vi "TdmsIcons_WriteIcon.vi"(8 "error in (no error)":errorcluster, 9 "Icon":T1, 10 "Function":string="Add", 11 "TdmsIn":refnum<k34>) -> (0 "error out":errorcluster, 3 "TdmsOut":refnum<k34>)   [LabVIEW 2014]
uses:
  <vilib>/picture/picture.llb/imagedata.ctl
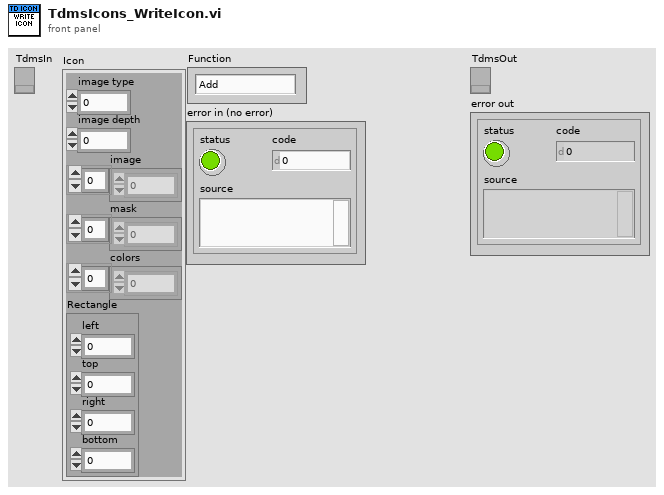
[diagram p1: front panel]
types:
  T1 = typedef "imagedata.ctl" = cluster{"image type":i32, "image depth":i32, "image":u8[], "mask":u8[], "colors":u32[], "Rectangle":cluster{"left":i16, "top":i16, "right":i16, "bottom":i16}}
  T2 = cluster{"left":i16, "top":i16, "right":i16, "bottom":i16}
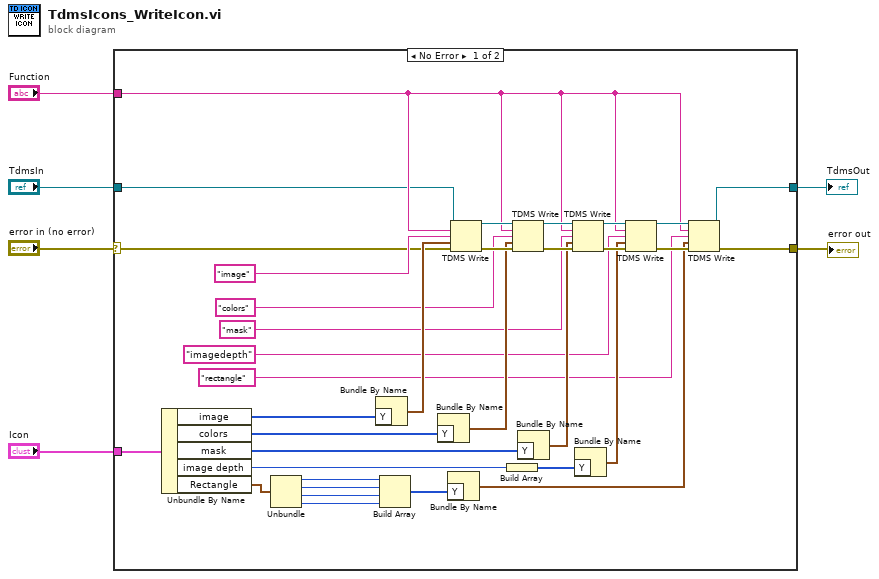
[diagram p0: block diagram]
diagram:
  n1 = case shown="No Error" "error in (no error)" {
    selector: "error in (no error)" -> [w9 w43]
    tunnel: "Function" -> [w22 _]
    tunnel: "TdmsIn" -> [w8 w42]
    tunnel: "Icon" -> [w11 _]
    tunnel: [w7 w42] -> w3
    tunnel: [w10 w43] -> w2
    frame No Error {
      n2 = Unbundle By Name(w11) -> ("image"=w40:u8[], "colors"=w37:u32[], "mask"=w36:u8[], "image depth"=w35:i32, "Rectangle"=w12:T2)
      n3 = Unbundle(w12) -> ("left"=w33:i16, "top"=w32:i16, "right"=w31:i16, "bottom"=w30:i16)
      n4 = Bundle By Name("Y"=w40) -> (w17:waveform(u8))  [unwired: 1 in]
      n5 = Build Array(w33, w32, w31, w30) -> (w29:i16[])
      n6 = Bundle By Name("Y"=w37) -> (w21:waveform(u32))  [unwired: 1 in]
      n7 = Bundle By Name("Y"=w29) -> (w18:waveform(i16))  [unwired: 1 in]
      n8 = TDMS Write(0:w8, 5:w22, 7:"image" ("group name in (Untitled)"), 9:w17, 11:w9) -> (4:w39:refnum<k34>, 15:w38:errorcluster)  [unwired: 1 in, 2 out]
      n9 = Build Array(w35) -> (w34:i32[])
      n10 = TDMS Write(0:w39, 5:w22, 7:"colors" ("group name in (Untitled)"), 9:w21, 11:w38) -> (4:w28:refnum<k34>, 15:w25:errorcluster)  [unwired: 1 in, 2 out]
      n11 = Bundle By Name("Y"=w36) -> (w20:waveform(u8))  [unwired: 1 in]
      n12 = TDMS Write(0:w28, 5:w22, 7:"mask" ("group name in (Untitled)"), 9:w20, 11:w25) -> (4:w27:refnum<k34>, 15:w26:errorcluster)  [unwired: 1 in, 2 out]
      n13 = Bundle By Name("Y"=w34) -> (w19:waveform(i32))  [unwired: 1 in]
      n14 = TDMS Write(0:w27, 5:w22, 7:"imagedepth" ("group name in (Untitled)"), 9:w19, 11:w26) -> (4:w24:refnum<k34>, 15:w23:errorcluster)  [unwired: 1 in, 2 out]
      n15 = TDMS Write(0:w24, 5:w22, 7:"rectangle" ("group name in (Untitled)"), 9:w18, 11:w23) -> (4:w7:refnum<k34>, 15:w10:errorcluster)  [unwired: 1 in, 2 out]
    }
    frame Error {
    }
  }
  "TdmsOut" <- w3
  "error out" <- w2
